vi "set_magnet_persitant.vi"   [LabVIEW 2019]
uses:
  Instrument_Setup.vi
  Global/Global Variables/Data_Display_global.vi
types:
  T1 = typedef "16T-Cluster.ctl" = cluster{"Clamp":bool, "Switch Heater":bool, "Go to Zero":bool, "Go to set":bool, "Go to Hold":bool, "Clamped":bool, "Quenched":bool, "Rate limit":bool, "Persistent":bool, "Hold":bool, "Set":bool, "Zero":bool, "Magnet (T)":dbl, "Leads (T)":dbl, "Magnet T (K)":dbl, "Switch":bool, "Setpoint (T)":dbl, "Rate (T/min)":dbl, "Select":bool, "Sweeping":bool}
  T2 = typedef "PSIO.ctl" = cluster{"Address":T3, "Version":enum16{"PS", "IPS"}}
  T3 = typedef "OxfordAddress.ctl" = cluster{"Com Port":i32, "ISOBUS Address":i32, "GPIB Address":i16, "Communication":enum16{"RS232", "ISOBUS", "GPIB", "Gateway"}}
  T4 = cluster{"Version\n":string, "Max Sweep(4.2K)":dbl[unit], "Max Sweep(2.2K)":dbl[unit], "Switch htr dly":dbl[unit], "Max Field(4.2K)":dbl[unit], "Max Field(2.2K)":dbl[unit], "Max lead res":dbl[unit], "IO Info":T2}
  T5 = typedef "15T-Cluster.ctl" = cluster{"Magnet (T)":dbl, "Leads (T)":dbl, "Setpoint (T)":dbl, "Rate (T/min)":dbl, "Set":bool, "Zero":bool, "Hold":bool, "Go to zero":bool, "Go to Hold":bool, "Go to Set":bool, "Clamp":bool, "Switch Heater":bool, "Rate limit":bool, "Switch":bool, "Clamped":bool, "Persistent":bool, "Quenched":bool, "Sweeping":bool, "Select":bool}
  T6 = cluster{"Version\n":string, "Max Sweep":dbl[unit], "Max Field":dbl[unit], "IO Info":T2, "Switch htr dly":dbl[unit]}
  T7 = typedef "P9_P14_Magnet-cluster.ctl" = cluster{"Magnet (Oe)":dbl, "Setpoint (Oe)":dbl, "Rate (Oe/min)":dbl, "Set Field":bool, "Go to zero":bool, "Set Persitant/non-pers":bool, "Approach":i32, "Magnet Status":i32, "Sweeping":bool, "Quenched":bool, "Persitant Mode ":bool, "Stable":bool, "Steps":dbl, "Paused Menu":dbl, "B Step Start Field":dbl}
  T8 = typedef "P9P14_Magnet_Control.ctl" = cluster{"Setpoint (Oe)":dbl, "Rate (Oe/min)":dbl, "Set Field":bool, "Go to zero":bool, "Set Persitant/non-pers":bool, "Approach":i32, "Steps":dbl, "Paused Menu":dbl, "B Step start Field":dbl}
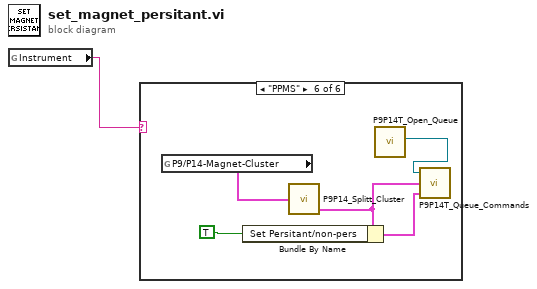
[diagram p0: block diagram]
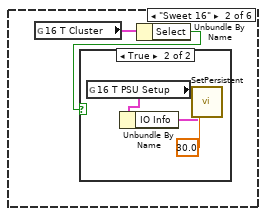
[diagram p3: hidden frame]
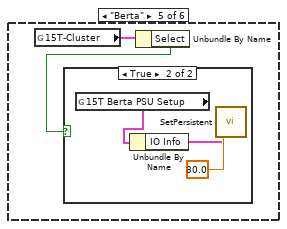
[diagram p7: hidden frame]
diagram:
  n1 = global read "Instrument_Setup.vi" "Instrument"() -> (w1:string)
  n2 = case shown="\"PPMS\"" w1 {
    frame "AMI", Default {
    }
    frame "Sweet 16" {
      n3 = global read "Data_Display_global.vi" "16 T Cluster"() -> (w3:T1)
      n4 = Unbundle By Name(w3) -> ("Select"=w2:bool)
      n5 = case shown="True" w2 {
        frame False {
        }
        frame True {
          n6 = global read "Instrument_Setup.vi" "16 T PSU Setup"() -> (w5:T4)
          n7 = Unbundle By Name(w5) -> ("IO Info"=w4:T2)
          n8 = call "SetPersistent.vi"("Switch Heater Dwell Time"=dbl[unit] 30.0, "IO Info"=w4) -> ()  [unwired: 1 in, 1 out]
        }
      }
    }
    frame "20T" {
    }
    frame "Mischer" {
    }
    frame "Berta" {
      n9 = global read "Data_Display_global.vi" "15T-Cluster"() -> (w8:T5)
      n10 = Unbundle By Name(w8) -> ("Select"=w7:bool)
      n11 = case shown="True" w7 {
        frame False {
        }
        frame True {
          n12 = global read "Instrument_Setup.vi" "15T Berta PSU Setup"() -> (w9:T6)
          n13 = Unbundle By Name(w9) -> ("IO Info"=w10:T2)
          n14 = call "SetPersistent.vi"("Switch Heater Dwell Time"=dbl[unit] 30.0, "IO Info"=w10) -> ()  [unwired: 1 in, 1 out]
        }
      }
    }
    frame "PPMS" {
      n15 = global read "Data_Display_global.vi" "P9/P14-Magnet-Cluster"() -> (w16:T7)
      n16 = call "P9P14_Splitt_Cluster.vi"("P9/P14-Magnet-Cluster"=w16) -> ("P9/P14-Magnet-Control"=w15:T8)  [unwired: 1 in, 1 out]
      n17 = Bundle By Name(cluster=w15, "Set Persitant/non-pers"=TRUE) -> (w13:T8)
      n18 = call "P9P14T_Open_Queue.vi"() -> ("queue out"=w12:refnum<queue>)  [unwired: 10 in, 1 out]
      n19 = call "P9P14T_Queue_Commands.vi"("P9/P14-Magnet-Control"=w13, "P9/P14-Magnet-Control old status"=w15, "16T Queue"=w12) -> ()  [unwired: 1 out]
    }
  }
